vi "Get Cursor Values from Data.vi"(7 "waveforms":T1, 10 "Refnums for FP Objects":T2, 11 "Display State In":T3={"Graph Visible Items"={"Plot Legend"=FALSE, "Scale Legend"=FALSE, "Graph Palette"=FALSE, "Cursor Legend"=FALSE, "X Scrollbar"=FALSE}, "View Table"=FALSE, "Table Visible Items"={"Vertical Scrollbar"=FALSE, "Horizontal Scrollbar"=FALSE, "Row Headers"=FALSE, "Column Headers"=FALSE, "Vertical Lines"=FALSE, "Horizontal Lines"=FALSE}, "Header Font"={"Font Name"="", "Size"=0, "Bold"=FALSE, "Italic"=FALSE, "Underline"=FALSE, "Strikeout"=FALSE, "Color"=0}, "Cell Font"={"Font Name"="", "Size"=0, "Bold"=FALSE, "Italic"=FALSE, "Underline"=FALSE, "Strikeout"=FALSE, "Color"=0}, "Description and Tip..."={"Description"="", "Tip"=""}, "Moveable Splitter Position"=0, "Measurement Cursor Configuration"={"relative to t0"={"enable relative time"=FALSE, "Relative times (DT)"=[], "color"=0}, "range"={"enable range"=FALSE, "T1"=0.0, "T2"=0.0, "Fixed interval (T2-T1)"=0.0, "T1 color"=0, "T2 color"=0, "enable shading"=FALSE}, "periodic"={"enable periodic"=FALSE, "First event (E1)"=0.0, "Number events (Ei)"=0, "Event spacing (s)"=0.0, "First color"=0, "Events color"=0}, "absolute timestamp"={"enable absolute"=FALSE, "Timestamps (TS)"=[], "color"=0}}, "X Increment"=0.0, "X Scale"={"Label Visible"=FALSE, "Label Text"="", "Time Mode"=enum."Relative", "Format String"=""}, "Y Scale"={"Label Visible"=FALSE, "Label Text"="", "Scaling"=enum."Engineering Units", "Format String"=""}, "Colors"={"background"=16777215, "major grid"=8355711, "minor grid"=12632256, "font"=0}, "Cursors"={"List"=[], "Tags"=[]}, "Plots"=[], "Plot Color Wheel"=[3381759, 32768, 982784, 4375295, 13827953, 13457919, 16757522, 4343295, 16728758, 12095254], "registered user events"=variant} caption="State") -> (2 "value table":string[][](array[string]), 3 "Display State Out":T3={"Graph Visible Items"={"Plot Legend"=FALSE, "Scale Legend"=FALSE, "Graph Palette"=FALSE, "Cursor Legend"=FALSE, "X Scrollbar"=FALSE}, "View Table"=FALSE, "Table Visible Items"={"Vertical Scrollbar"=FALSE, "Horizontal Scrollbar"=FALSE, "Row Headers"=FALSE, "Column Headers"=FALSE, "Vertical Lines"=FALSE, "Horizontal Lines"=FALSE}, "Header Font"={"Font Name"="", "Size"=0, "Bold"=FALSE, "Italic"=FALSE, "Underline"=FALSE, "Strikeout"=FALSE, "Color"=0}, "Cell Font"={"Font Name"="", "Size"=0, "Bold"=FALSE, "Italic"=FALSE, "Underline"=FALSE, "Strikeout"=FALSE, "Color"=0}, "Description and Tip..."={"Description"="", "Tip"=""}, "Moveable Splitter Position"=0, "Measurement Cursor Configuration"={"relative to t0"={"enable relative time"=FALSE, "Relative times (DT)"=[], "color"=0}, "range"={"enable range"=FALSE, "T1"=0.0, "T2"=0.0, "Fixed interval (T2-T1)"=0.0, "T1 color"=0, "T2 color"=0, "enable shading"=FALSE}, "periodic"={"enable periodic"=FALSE, "First event (E1)"=0.0, "Number events (Ei)"=0, "Event spacing (s)"=0.0, "First color"=0, "Events color"=0}, "absolute timestamp"={"enable absolute"=FALSE, "Timestamps (TS)"=[], "color"=0}}, "X Increment"=0.0, "X Scale"={"Label Visible"=FALSE, "Label Text"="", "Time Mode"=enum."Relative", "Format String"=""}, "Y Scale"={"Label Visible"=FALSE, "Label Text"="", "Scaling"=enum."Engineering Units", "Format String"=""}, "Colors"={"background"=16777215, "major grid"=8355711, "minor grid"=12632256, "font"=0}, "Cursors"={"List"=[], "Tags"=[]}, "Plots"=[], "Plot Color Wheel"=[3381759, 32768, 982784, 4375295, 13827953, 13457919, 16757522, 4343295, 16728758, 12095254], "registered user events"=variant} caption="State", 4 "measurement names":string[](array[string]), 5 "waveforms":T1, 6 "channels":string[](array[string]))   [LabVIEW 2017, in "Waveforms with Cursors.xctl"]
doc: "This VI extracts the spectral values at the cursor positions. Based on the spectral data, Row Headers, Column Headers, and Values are written to the table."
uses:
  <vilib>/addons/_XControls/Waveforms with Cursors/Waveforms with Cursors.xctl
  <vilib>/addons/_XControls/Waveforms with Cursors/Controls/State.ctl
  <vilib>/Utility/miscctls.llb/LVFontTypeDef.ctl
  <vilib>/addons/_XControls/Waveforms with Cursors/Controls/Waveform Cursor Configuration.ctl
  <vilib>/addons/_XControls/Waveforms with Cursors/Controls/Data.ctl
  <vilib>/addons/_XControls/Waveforms with Cursors/Controls/Refnums Typedef.ctl
  <vilib>/addons/_NISVFA/_Shared subVIs/Common/svc_Coerce Index and Length.vi
  <vilib>/addons/_NISVFA/_Shared subVIs/Common/svc_Conditional Merge Error.vi
  <vilib>/Waveform/WDTOps.llb/WDT Get XY Value DBL.vi
  <vilib>/addons/_NISVFA/_Shared subVIs/Common/svc_Engineering Units to Unit Label.vi
  <vilib>/addons/_NISVFA/_Shared subVIs/Common/svc_Unit Label to Engineering Units.vi
  <vilib>/Analysis/NI_AALBase.lvlib
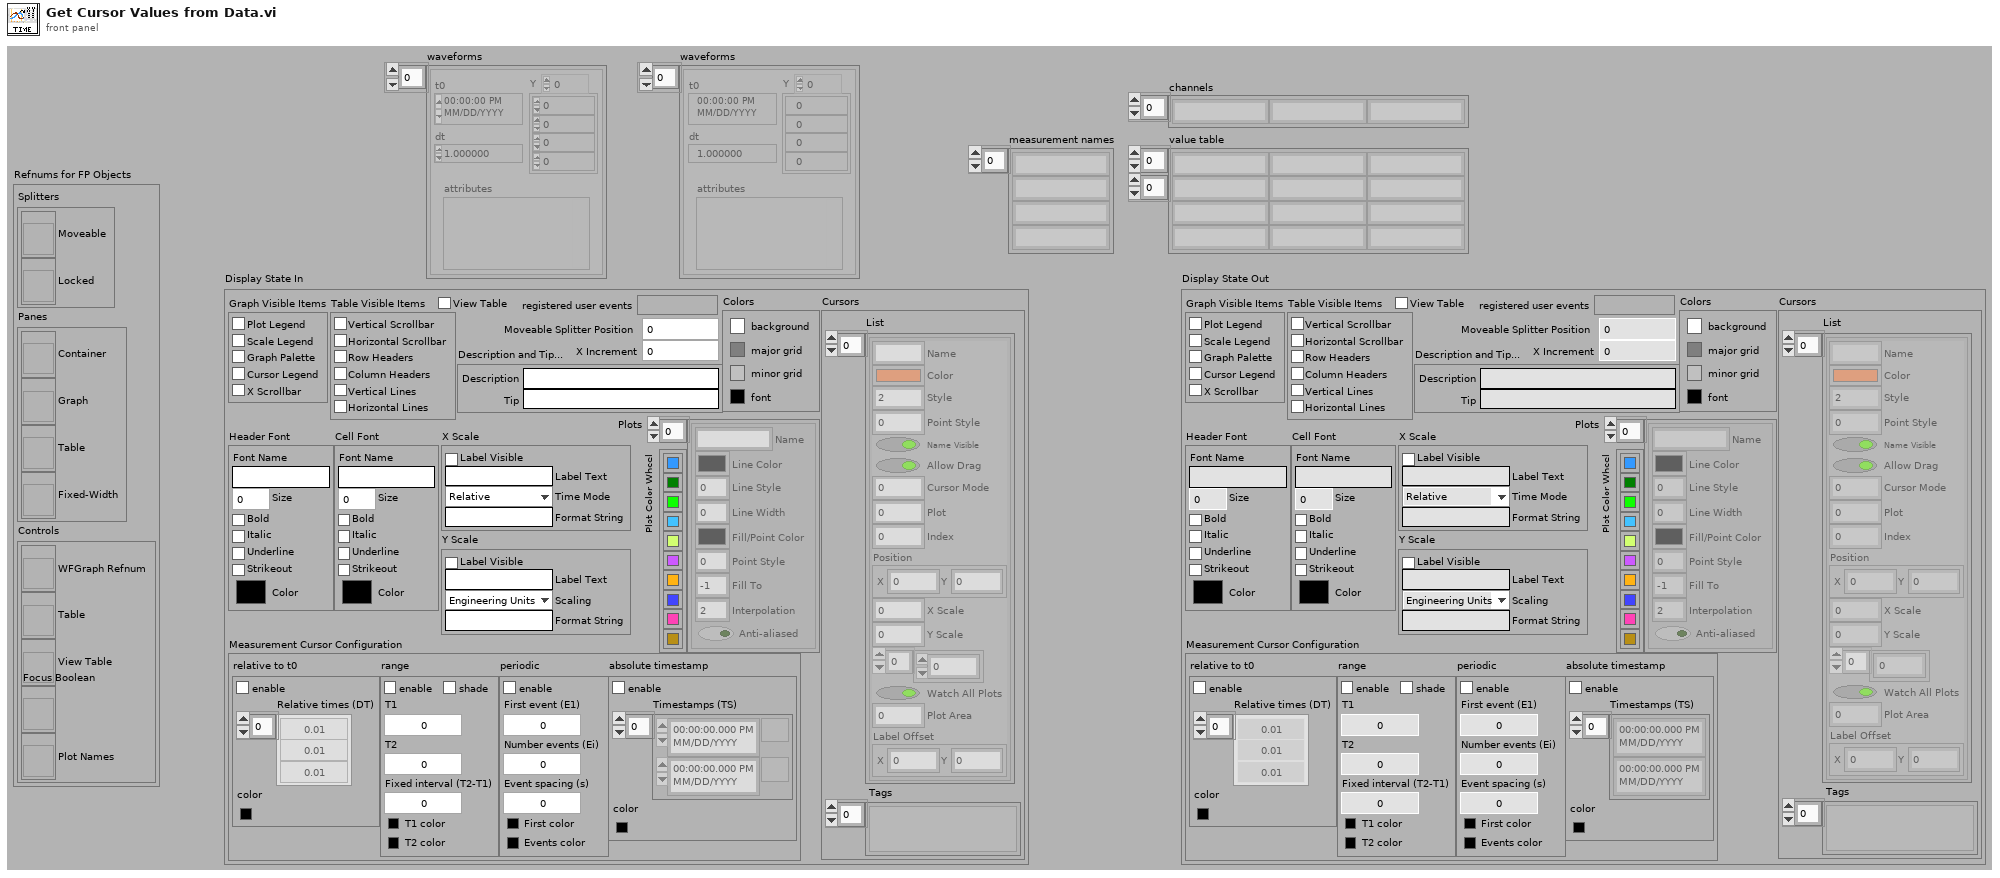
[diagram p1: front panel]
types:
  T1 = typedef "Waveforms with Cursors.xctl/Data.ctl" = waveform(dbl)[]
  T2 = typedef "Waveforms with Cursors.xctl/Refnums Typedef.ctl" = cluster{"Splitters":cluster{"Moveable":refnum<vi>, "Locked":refnum<vi>}, "Panes":cluster{"Container":refnum<vi>, "Graph":refnum<vi>, "Table":refnum<vi>, "Fixed-Width":refnum<vi>}, "Controls":cluster{"WFGraph Refnum":refnum<vi>, "Table":refnum<vi>, "View Table":refnum<vi>, "Focus Boolean":refnum<vi>, "Plot Names":refnum<vi>}}
  T3 = typedef "Waveforms with Cursors.xctl/State.ctl" = cluster{"Graph Visible Items":cluster{"Plot Legend":bool, "Scale Legend":bool, "Graph Palette":bool, "Cursor Legend":bool, "X Scrollbar":bool}, "View Table":bool, "Table Visible Items":cluster{"Vertical Scrollbar":bool, "Horizontal Scrollbar":bool, "Row Headers":bool, "Column Headers":bool, "Vertical Lines":bool, "Horizontal Lines":bool}, "Header Font":T4, "Cell Font":T4, "Description and Tip...":cluster{"Description":string, "Tip":string}, "Moveable Splitter Position":i32, "Measurement Cursor Configuration":T5, "X Increment":dbl, "X Scale":cluster{"Label Visible":bool, "Label Text":string, "Time Mode":enum16{"Relative", "Absolute"}, "Format String":string}, "Y Scale":cluster{"Label Visible":bool, "Label Text":string, "Scaling":enum16{"Engineering Units", "Voltage"}, "Format String":string}, "Colors":cluster{"background":u32, "major grid":u32, "minor grid":u32, "font":u32}, "Cursors":cluster{"List":cluster{"Name":string, "Color":u32, "Style":i32, "Point Style":u8, "Name Visible":bool, "Allow Drag":bool, "Cursor Mode":u32, "Plot":i32, "Index":i32, "Position":cluster{"X":dbl, "Y":dbl}, "X Scale":u32, "Y Scale":u32, "Watch Plots":i32[], "Watch All Plots":bool, "Plot Area":i32, "Label Offset":cluster{"X":dbl, "Y":dbl}}[], "Tags":variant[]}, "Plots":cluster{"Name":string, "Line Color":u32, "Line Style":u8, "Line Width":u8, "Fill/Point Color":u32, "Point Style":u8, "Fill To":i16, "Interpolation":u8, "Anti-aliased":bool}[], "Plot Color Wheel":u32[], "registered user events":variant}
  T4 = typedef "LVFontTypeDef.ctl" = cluster{"Font Name":string, "Size":u16, "Bold":bool, "Italic":bool, "Underline":bool, "Strikeout":bool, "Color":u32}
  T5 = typedef "Waveforms with Cursors.xctl/Waveform Cursor Configuration.ctl" = cluster{"relative to t0":cluster{"enable relative time":bool, "Relative times (DT)":dbl[], "color":u32}, "range":cluster{"enable range":bool, "T1":dbl, "T2":dbl, "Fixed interval (T2-T1)":dbl, "T1 color":u32, "T2 color":u32, "enable shading":bool}, "periodic":cluster{"enable periodic":bool, "First event (E1)":dbl, "Number events (Ei)":i32, "Event spacing (s)":dbl, "First color":u32, "Events color":u32}, "absolute timestamp":cluster{"enable absolute":bool, "Timestamps (TS)":timestamp[], "color":u32}}
  T6 = cluster{"List":cluster{"Name":string, "Color":u32, "Style":i32, "Point Style":u8, "Name Visible":bool, "Allow Drag":bool, "Cursor Mode":u32, "Plot":i32, "Index":i32, "Position":cluster{"X":dbl, "Y":dbl}, "X Scale":u32, "Y Scale":u32, "Watch Plots":i32[], "Watch All Plots":bool, "Plot Area":i32, "Label Offset":cluster{"X":dbl, "Y":dbl}}[], "Tags":variant[]}
  T7 = cluster{"Name":string, "Color":u32, "Style":i32, "Point Style":u8, "Name Visible":bool, "Allow Drag":bool, "Cursor Mode":u32, "Plot":i32, "Index":i32, "Position":cluster{"X":dbl, "Y":dbl}, "X Scale":u32, "Y Scale":u32, "Watch Plots":i32[], "Watch All Plots":bool, "Plot Area":i32, "Label Offset":cluster{"X":dbl, "Y":dbl}}[]
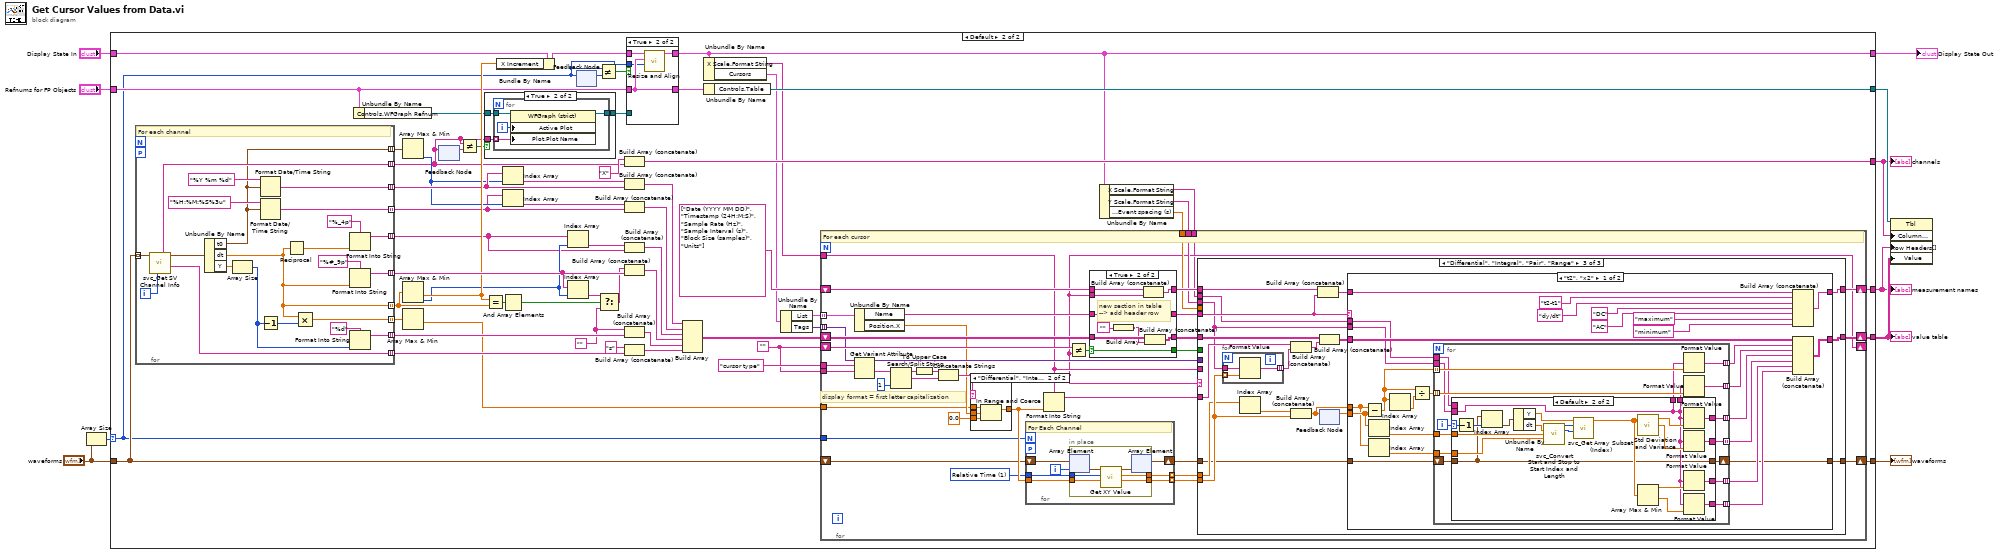
[diagram p0: block diagram]
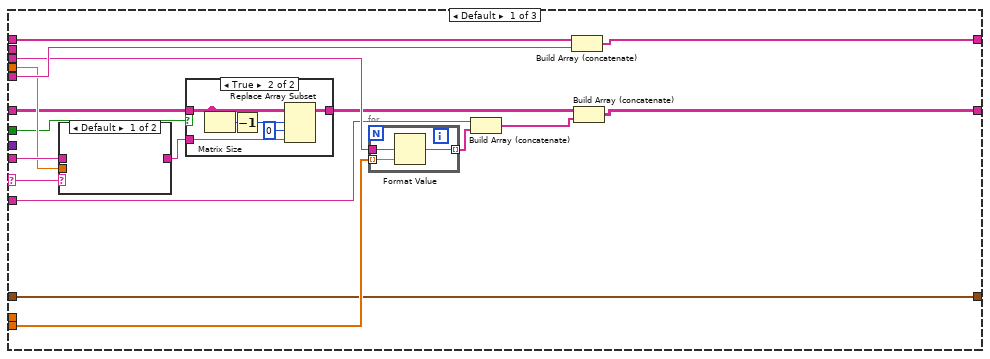
[diagram p7: hidden frame]
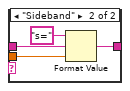
[diagram p9: hidden frame]
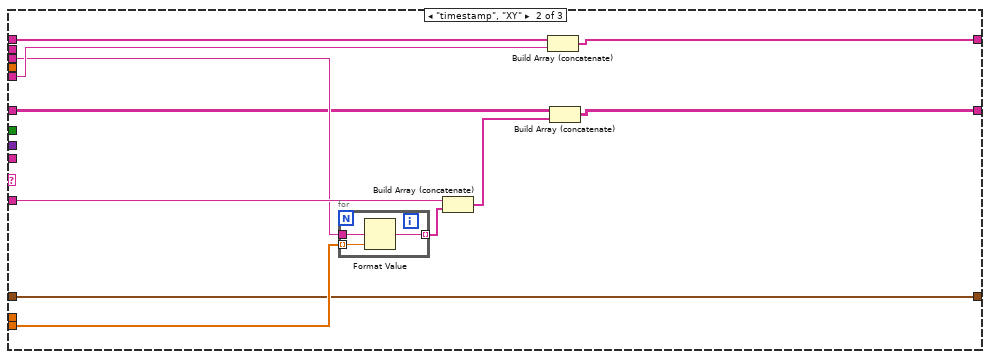
[diagram p10: hidden frame]
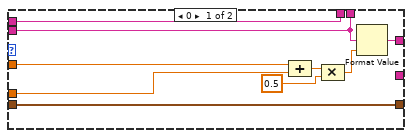
[diagram p11: hidden frame]
diagram:
  n1 = Array Size(array="waveforms") -> (size(s)=w6:i32)
  n2 = case shown="Default" w6 {
    selector: w6 -> [_ w16]
    tunnel: [_ w67] -> w3
    tunnel: [_ w66] -> w2
    tunnel: [_ w65] -> w4
    tunnel: [w14 w45] -> w10
    tunnel: "waveforms" -> [w11 w60]
    tunnel: "Display State In" -> [w14 w47]
    tunnel: "Refnums for FP Objects" -> [w13 w44]
    tunnel: [w12 w49] -> w5
    tunnel: [w11 w15] -> w1
    frame 0 {
      n3 = Unbundle By Name(w13) -> ("Controls.Table"=w12:refnum<vi>)
    }
    frame Default {
      w64 = "" ("String")
      w27 = "" ("String")
      n4 = for {
        tunnel: [w105] -> w18 mode=indexing
        tunnel: w60 -> [w107] mode=indexing
        tunnel: [w104] -> w73 mode=indexing
        tunnel: [w109] -> w58 mode=indexing
        tunnel: [w108] -> w54 mode=indexing
        tunnel: [w90] -> w55 mode=indexing
        tunnel: [w100] -> w40 mode=indexing
        tunnel: [w99] -> w37 mode=indexing
        tunnel: [w98] -> w34 mode=indexing
        tunnel: [w95] -> w29 mode=indexing
        tunnel: [w88] -> w21 mode=indexing
        workers-P: _ -> [_]
        i -> [w103]
        # "For each channel"
        n5 = call <vilib>:"svc_Get SV Channel Info.vi"("channel index"=w103, "scaled signal [EU]"=w107) -> ("unit label"=w104:string, "dup scaled signal [EU]"=w106:waveform(dbl), "channel name"=w105:string)  [unwired: 4 in, 3 out]
        n6 = Unbundle By Name(w106) -> ("t0"=w100:timestamp, "dt"=w90:dbl, "Y"=w93:dbl[])
        n7 = Array Size(array=w93) -> (size(s)=w89:i32)
        n8 = Format Date/Time String(time format string (%c)="%Y %m %d" ("format string"), seconds (now)=w100) -> (date/time string=w99:string)  [unwired: 1 in]
        n9 = Format Date/Time String(time format string (%c)="%H:%M:%S%3u" ("format string"), seconds (now)=w100) -> (date/time string=w98:string)  [unwired: 1 in]
        n10 = Decrement(x=w89) -> (x-1=w91:i32)
        n11 = Reciprocal(x=w90) -> (1/x=w97:dbl)
        n12 = Multiply(x=w90, y=w91) -> (x*y=w88:dbl)
        n13 = Format Into String(format string="%_4p", w97) -> (resulting string=w95:string)  [unwired: 2 in, 1 out]
        n14 = Format Into String(format string="%#_9p", w90) -> (resulting string=w109:string)  [unwired: 2 in, 1 out]
        n15 = Format Into String(format string="%d", w89) -> (resulting string=w108:string)  [unwired: 2 in, 1 out]
      }
      n16 = Unbundle By Name(w44) -> ("Controls.WFGraph Refnum"=w50:refnum<vi>)
      n17 = Array Max & Min(array=w40) -> (min index (indices)=w36:i32)  [unwired: 3 out]
      n18 = Array Max & Min(array=w55) -> (min value=w56:dbl, min index (indices)=w31:i32)  [unwired: 2 out]
      n19 = Array Max & Min(array=w21) -> (min value=w20:dbl)  [unwired: 3 out]
      n20 = feedback-in #1(w18) -> ()
      n21 = feedback #1() -> (w19:string[])  [unwired: 1 in]
      n22 = Not Equal?(x=w18, y=w19) -> (x != y?=w17:bool)
      n23 = case shown="True" w17 {
        tunnel: w50 -> [w74 w77]
        tunnel: w18 -> [_ w76]
        tunnel: [w74 w75] -> w41
        frame False {
        }
        frame True {
          n24 = for {
            tunnel: w77 -> [w81]
            tunnel: w76 -> [w79] mode=indexing
            tunnel: [w78] -> w75
            i -> [w80]
            n25 = property class="WFGraph (strict)"(reference=w81, "Active Plot"=w80, "Plot.Plot Name"=w79) -> (reference out=w78:refnum<vi>)  [unwired: 1 in, 1 out]
          }
        }
      }
      n26 = Equal?(x=w56, y=w55) -> (x = y?=w57:bool[])
      n27 = Bundle By Name(cluster=w47, "X Increment"=w56) -> (w46:T3)
      n28 = Index Array(array=w37, index=w36) -> (element=w38:string)
      n29 = Index Array(array=w34, index=w36) -> (element=w35:string)
      n30 = And Array Elements(Boolean array=w57) -> (logical AND=w53:bool)
      n31 = Index Array(array=w29, index=w31) -> (element=w30:string)
      n32 = Index Array(array=w58, index=w31) -> (element=w52:string)
      n33 = feedback #2() -> (w59:i32)  [unwired: 1 in]
      n34 = feedback-in #2(w16) -> ()
      n35 = Not Equal?(x=w16, y=w59) -> (x != y?=w42:bool)
      n36 = Select(t=w52, s=w53, f=w27) -> (s? t:f=w51:string)
      n37 = Build Array (concatenate)("X" ("String"), w18) -> (w65:string[])
      n38 = Build Array (concatenate)(w38, w37) -> (w32:string[])
      n39 = Build Array (concatenate)(w35, w34) -> (w33:string[])
      n40 = Build Array (concatenate)(w30, w29) -> (w28:string[])
      n41 = Build Array (concatenate)(w51, w58) -> (w68:string[])
      n42 = Build Array (concatenate)(w27, w54) -> (w71:string[])
      n43 = Build Array (concatenate)("s" ("x-axis unit label"), w73) -> (w72:string[])
      n44 = case shown="True" w42 {
        tunnel: w46 -> [w83 w87]
        tunnel: [w83 w86] -> w45
        tunnel: w44 -> [w82 w85]
        tunnel: [w82 w85] -> w43
        tunnel: w16 -> [_ w84]
        tunnel: w41 -> [_ _]
        frame False {
        }
        frame True {
          n45 = call <vilib>:"Resize and Align.vi"("number of channels"=w84, "Refnums for Resizing and Alignment"=w85, "State in"=w87) -> ("State out"=w86:T3)  [unwired: 7 in, 1 out]
        }
      }
      n46 = Build Array(w32, w33, w28, w68, w71, w72) -> (w62:string[][])
      n47 = Unbundle By Name(w45) -> ("X Scale.Format String"=w48:string, "Cursors"=w24:T6)
      n48 = Unbundle By Name(w43) -> ("Controls.Table"=w49:refnum<vi>)
      n49 = Unbundle By Name(w24) -> ("List"=w23:T7, "Tags"=w25:variant[])
      n50 = Unbundle By Name(w45) -> ("X Scale.Format String"=w22:string, "Y Scale.Format String"=w63:string, "Measurement Cursor Configuration.periodic.Event spacing (s)"=w61:dbl)
      n51 = for {
        shift-right: [w147] -> w66
        shift-left: string[] ["Date (YYYY MM DD)", "Timestamp (24H:M:S)", "Sample Rate (Hz)", "Sample Interval (s)", "Block Size (samples)", "Units"] ("Array") -> [w138]
        shift-right: [w146] -> w67
        shift-left: w62 -> [w139]
        tunnel: "cursor type" -> [w145]
        shift-right: [w124] -> _
        shift-left: w64 -> [w144]
        tunnel: w64 -> [w143]
        tunnel: w48 -> [w126]
        tunnel: w63 -> [w128]
        tunnel: w61 -> [w125]
        tunnel: w20 -> [w122]
        tunnel: w25 -> [w114] mode=indexing
        tunnel: w23 -> [w113] mode=indexing
        tunnel: w22 -> [w112]
        tunnel: w16 -> [w111]
        shift-right: [w110] -> w15
        shift-left: w60 -> [w119]
        w115 = u16 1 items=["Samples", "Relative Time"] ("Y position format")
        # "display format = first letter capitalization"
        # "For each cursor"
        n52 = Unbundle By Name(w113) -> ("Name"=w140:string, "Position.X"=w123:dbl)
        n53 = Get Variant Attribute(Variant=w114, name=w145, default value (empty Variant)=w143) -> (duplicate Variant=w130:variant, value=w131:string)  [unwired: 1 in, 2 out]
        n54 = Search/Split String(string=w131, offset (0)=1) -> (substring before match=w134:string, match + rest of string=w132:string)  [unwired: 1 in, 1 out]
        n55 = To Upper Case(1:w134) -> (0:w133:string)
        n56 = Concatenate Strings(w133, w132) -> (w124:string)
        n57 = case shown="\"Differential\", \"Integral\", \"Pair\", \"Range\"" w124 {
          tunnel: w123 -> [w161 w165]
          tunnel: [w161 w164] -> w120
          tunnel: 0.0 -> [_ w163]
          tunnel: w122 -> [_ w162]
          frame Default {
          }
          frame "Differential", "Integral", "Pair", "Range" {
            n58 = In Range and Coerce(upper limit=w162, x=w165, lower limit=w163) -> (coerced(x)=w164:dbl)  [unwired: 1 out]
          }
        }
        n59 = for {
          N: w111 -> [_]
          tunnel: w120 -> [w154]
          tunnel: [w153] -> w117 mode=indexing
          tunnel: [w152] -> w116 mode=indexing
          tunnel: w115 -> [w151]
          workers-P: _ -> [_]
          shift-right: [w148] -> w118
          shift-left: w119 -> [w149]
          i -> [w150]
          # "For Each Channel"
          n60 = in-place {
            in-place-border: w154 -> [w160]
            in-place-border: [w159] -> w153
            in-place-border: [w158] -> w152
            in-place-border: w151 -> [w157]
            n61 = in-place-array #3(w149, w150) -> (w156:waveform(dbl))
            n62 = call-poly <vilib>:"Get XY Value.vi"("Y position"=w160, "Y position format"=w157, "waveform in"=w156) -> ("Y value"=w159:dbl, "actual Y position"=w158:dbl, "waveform out"=w155:waveform(dbl))  [unwired: 4 in, 2 out]
            n63 = in-place-array #3(w155) -> (w148:T1)  [unwired: 1 out]
          }
        }
        n64 = Format Into String(format string=w126, w120) -> (resulting string=w129:string)  [unwired: 2 in, 1 out]
        n65 = Not Equal?(x=w144, y=w124) -> (x != y?=w142:bool)
        n66 = case shown="True" w142 {
          selector: w142 -> [w166 w170]
          tunnel: [w169 w178] -> w141
          tunnel: w140 -> [w169 w178]
          tunnel: w139 -> [w167 w173]
          tunnel: w138 -> [w168 w176]
          tunnel: [w168 w177] -> w137
          tunnel: [w167 w174] -> w136
          tunnel: w124 -> [_ w175]
          tunnel: [w166 w170] -> w127
          frame False {
          }
          frame True {
            # "new section in table\n--> add header row"
            n67 = Build Array("") -> (w171:string[])
            n68 = Build Array (concatenate)(w176, w175) -> (w177:string[])
            n69 = Build Array (concatenate)(w173, w171) -> (w174:string[][])
          }
        }
        n70 = case shown="\"Differential\", \"Integral\", \"Pair\", \"Range\"" w124 {
          selector: w124 -> [w187 _ _]
          tunnel: w117 -> [w189 w216 w237]
          tunnel: w137 -> [w195 w220 w242]
          tunnel: w141 -> [w194 w219 w236]
          tunnel: [w193 w218 w235] -> w147
          tunnel: w136 -> [w183 w211 w241]
          tunnel: [w192 w217 w232] -> w146
          tunnel: w130 -> [_ _ _]
          tunnel: w129 -> [w186 w215 w239]
          tunnel: w128 -> [w190 w212 w227]
          tunnel: w127 -> [w181 _ _]
          tunnel: w126 -> [w185 _ _]
          tunnel: w125 -> [w184 _ _]
          tunnel: w116 -> [_ _ w231]
          tunnel: w118 -> [w179 w210 w226]
          tunnel: w112 -> [_ _ w225]
          tunnel: [w179 w210 w224] -> w110
          frame Default {
            n71 = case shown="Default" w187 {
              tunnel: w185 -> [_ w205]
              tunnel: w184 -> [_ w204]
              tunnel: [_ w203] -> w180
              frame Default {
              }
              frame "Sideband" {
                n72 = Format Value(string ("")="s=", format string=w205, value (0)=w204) -> (output string=w203:string)
              }
            }
            n73 = case shown="True" w181 {
              tunnel: w183 -> [w196 w200]
              tunnel: [w196 w202] -> w182
              tunnel: w180 -> [_ w198]
              frame False {
              }
              frame True {
                n74 = Matrix Size(0:w200) -> (1:w201:i32)  [unwired: 1 out]
                n75 = Decrement(x=w201) -> (x-1=w199:i32)
                n76 = Replace Array Subset(array=w200, new element=w198, index (row)=w199, index (col)=0 ("disabled index (col)")) -> (w202:string[][])
              }
            }
            n77 = for {
              tunnel: w189 -> [w209] mode=indexing
              tunnel: [w208] -> w191 mode=indexing
              tunnel: w190 -> [w207]
              n78 = Format Value(format string=w207, value (0)=w209) -> (output string=w208:string)  [unwired: 1 in]
            }
            n79 = Build Array (concatenate)(w186, w191) -> (w188:string[])
            n80 = Build Array (concatenate)(w195, w194) -> (w193:string[])
            n81 = Build Array (concatenate)(w182, w188) -> (w192:string[][])
          }
          frame "timestamp", "XY" {
            n82 = for {
              tunnel: w216 -> [w223] mode=indexing
              tunnel: [w222] -> w213 mode=indexing
              tunnel: w212 -> [w221]
              n83 = Format Value(format string=w221, value (0)=w223) -> (output string=w222:string)  [unwired: 1 in]
            }
            n84 = Build Array (concatenate)(w215, w213) -> (w214:string[])
            n85 = Build Array (concatenate)(w220, w219) -> (w218:string[])
            n86 = Build Array (concatenate)(w211, w214) -> (w217:string[][])
          }
          frame "Differential", "Integral", "Pair", "Range" {
            n87 = for {
              tunnel: w237 -> [w321] mode=indexing
              tunnel: [w320] -> w240 mode=indexing
              tunnel: w227 -> [w319]
              n88 = Format Value(format string=w319, value (0)=w321) -> (output string=w320:string)  [unwired: 1 in]
            }
            n89 = Index Array(array=w231) -> (element=w230:dbl)  [unwired: 1 in]
            n90 = Build Array (concatenate)(w239, w240) -> (w238:string[])
            n91 = Build Array (concatenate)(w230, w237) -> (w229:dbl[])
            n92 = Build Array (concatenate)(w242, w236) -> (w234:string[])
            n93 = Build Array (concatenate)(w241, w238) -> (w233:string[][])
            n94 = feedback-in #4(w229) -> ()
            n95 = feedback #4() -> (w228:dbl[])  [unwired: 1 in]
            n96 = case shown="\"t2\", \"x2\"" w236 {
              tunnel: [w252 w318] -> w235
              tunnel: w234 -> [w269 w318]
              tunnel: w233 -> [w267 w317]
              tunnel: [w251 w317] -> w232
              tunnel: w229 -> [w259 _]
              tunnel: w228 -> [w260 _]
              tunnel: w227 -> [w245 _]
              tunnel: w226 -> [w254 w316]
              tunnel: w225 -> [w244 _]
              tunnel: [w243 w316] -> w224
              frame "t2", "x2" {
                n97 = Subtract(x=w259, y=w260) -> (x-y=w264:dbl[])
                n98 = Index Array(array=w260) -> (element=w256:dbl)  [unwired: 1 in]
                n99 = Index Array(array=w259) -> (element=w255:dbl)  [unwired: 1 in]
                n100 = Index Array(array=w264) -> (element=w265:dbl)  [unwired: 1 in]
                n101 = Divide(x=w264, y=w265) -> (x/y=w263:dbl[])
                n102 = for {
                  tunnel: w264 -> [w286] mode=indexing
                  tunnel: [w285] -> w266 mode=indexing
                  tunnel: w263 -> [w284] mode=indexing
                  tunnel: [w283] -> w262 mode=indexing
                  tunnel: [w280] -> w250 mode=indexing
                  tunnel: [w279] -> w258 mode=indexing
                  tunnel: w256 -> [w278]
                  tunnel: w255 -> [w277]
                  tunnel: [w275] -> w247 mode=indexing
                  tunnel: [w274] -> w246 mode=indexing
                  tunnel: w245 -> [w273]
                  tunnel: w244 -> [w271]
                  shift-right: [w270] -> w243
                  shift-left: w254 -> [w276]
                  i -> [w282]
                  n103 = case shown="Default" w282 {
                    selector: w282 -> [_ w315]
                    tunnel: [w289 w298] -> w281
                    tunnel: [_ w314] -> w280
                    tunnel: [w292 w313] -> w279
                    tunnel: w278 -> [w291 w309]
                    tunnel: w277 -> [w290 w308]
                    tunnel: w276 -> [w287 w296]
                    tunnel: [_ w301] -> w275
                    tunnel: [_ w300] -> w274
                    tunnel: w273 -> [w289 w298]
                    tunnel: [w288 w298] -> w272
                    tunnel: w271 -> [w288 _]
                    tunnel: [w287 w296] -> w270
                    frame 0 {
                      n104 = Compound Arithmetic op=ADD(w291, w290) -> (w295:dbl)
                      n105 = Compound Arithmetic op=MULTIPLY(w295, 0.5 ("value")) -> (w293:dbl)
                      n106 = Format Value(format string=w289, value (0)=w293) -> (output string=w292:string)  [unwired: 1 in]
                    }
                    frame Default {
                      n107 = Decrement(x=w315) -> (x-1=w310:i32)
                      n108 = Index Array(array=w296, index=w310) -> (element=w307:waveform(dbl))
                      n109 = Unbundle By Name(w307) -> ("Y"=w299:dbl[], "dt"=w311:dbl)
                      n110 = call <vilib>:"svc_Convert Start and Stop to Start Index and Length.vi"("df"=w311, "start frequency"=w309, "stop frequency"=w308) -> ("start index"=w312:i32, "band length"=w306:i32)  [unwired: 9 in, 2 out]
                      n111 = call <vilib>:"svc_Get Array Subset (Index).vi"("length (-1 = all)"=w306, "start index (0)"=w312, "Y"=w299) -> ("Y subset"=w297:dbl[])  [unwired: 4 in, 4 out]
                      n112 = call <vilib>:"Std Deviation and Variance.vi"("X"=w297) -> ("mean"=w305:dbl, "standard deviation"=w302:dbl)  [unwired: 1 in, 1 out]
                      n113 = Array Max & Min(array=w297) -> (max value=w303:dbl, min value=w304:dbl)  [unwired: 2 out]
                      n114 = Format Value(format string=w298, value (0)=w305) -> (output string=w313:string)  [unwired: 1 in]
                      n115 = Format Value(format string=w298, value (0)=w302) -> (output string=w314:string)  [unwired: 1 in]
                      n116 = Format Value(format string=w298, value (0)=w303) -> (output string=w301:string)  [unwired: 1 in]
                      n117 = Format Value(format string=w298, value (0)=w304) -> (output string=w300:string)  [unwired: 1 in]
                    }
                  }
                  n118 = Format Value(format string=w272, value (0)=w286) -> (output string=w285:string)  [unwired: 1 in]
                  n119 = Format Value(format string=w281, value (0)=w284) -> (output string=w283:string)  [unwired: 1 in]
                }
                n120 = Build Array (concatenate)(w269, "t2-t1", "dy/dt", "DC", "AC", "maximum", "minimum") -> (w252:string[])
                n121 = Build Array (concatenate)(w267, w266, w262, w258, w250, w247, w246) -> (w251:string[][])
              }
              frame "t1", "x1", Default {
              }
            }
          }
        }
      }
    }
  }
  "channels" <- w4
  "measurement names" <- w2
  "value table" <- w3
  "Display State Out" <- w10
  "waveforms" <- w1
  n122 = property class="Tbl"(reference=w5, "Column Headers[]"=w4, "Row Headers[]"=w2, "Value"=w3) -> ()  [unwired: 1 in, 2 out]
